vi "AB_Engine_AddExportClassInfo.vi"(8 "ClassInfo":T1[](array[typedef]), 10 "DataTypes":string[](array[string]), 11 "ExportClassInfo":T1[](array[typedef])) -> (3 "ExportClassInfoOut":T1[](array[typedef]))   [LabVIEW 2020]
uses:
  <vilib>/AppBuilder/AB_InteropAssembly_DistVI_Class_Info.ctl
  <vilib>/AppBuilder/IOStatus.ctl
  <vilib>/xml/Close Reference(Node).vi
  <vilib>/xml/NI_XML.lvlib
  <resource>/objmgr/DOMUserDefRef.rc
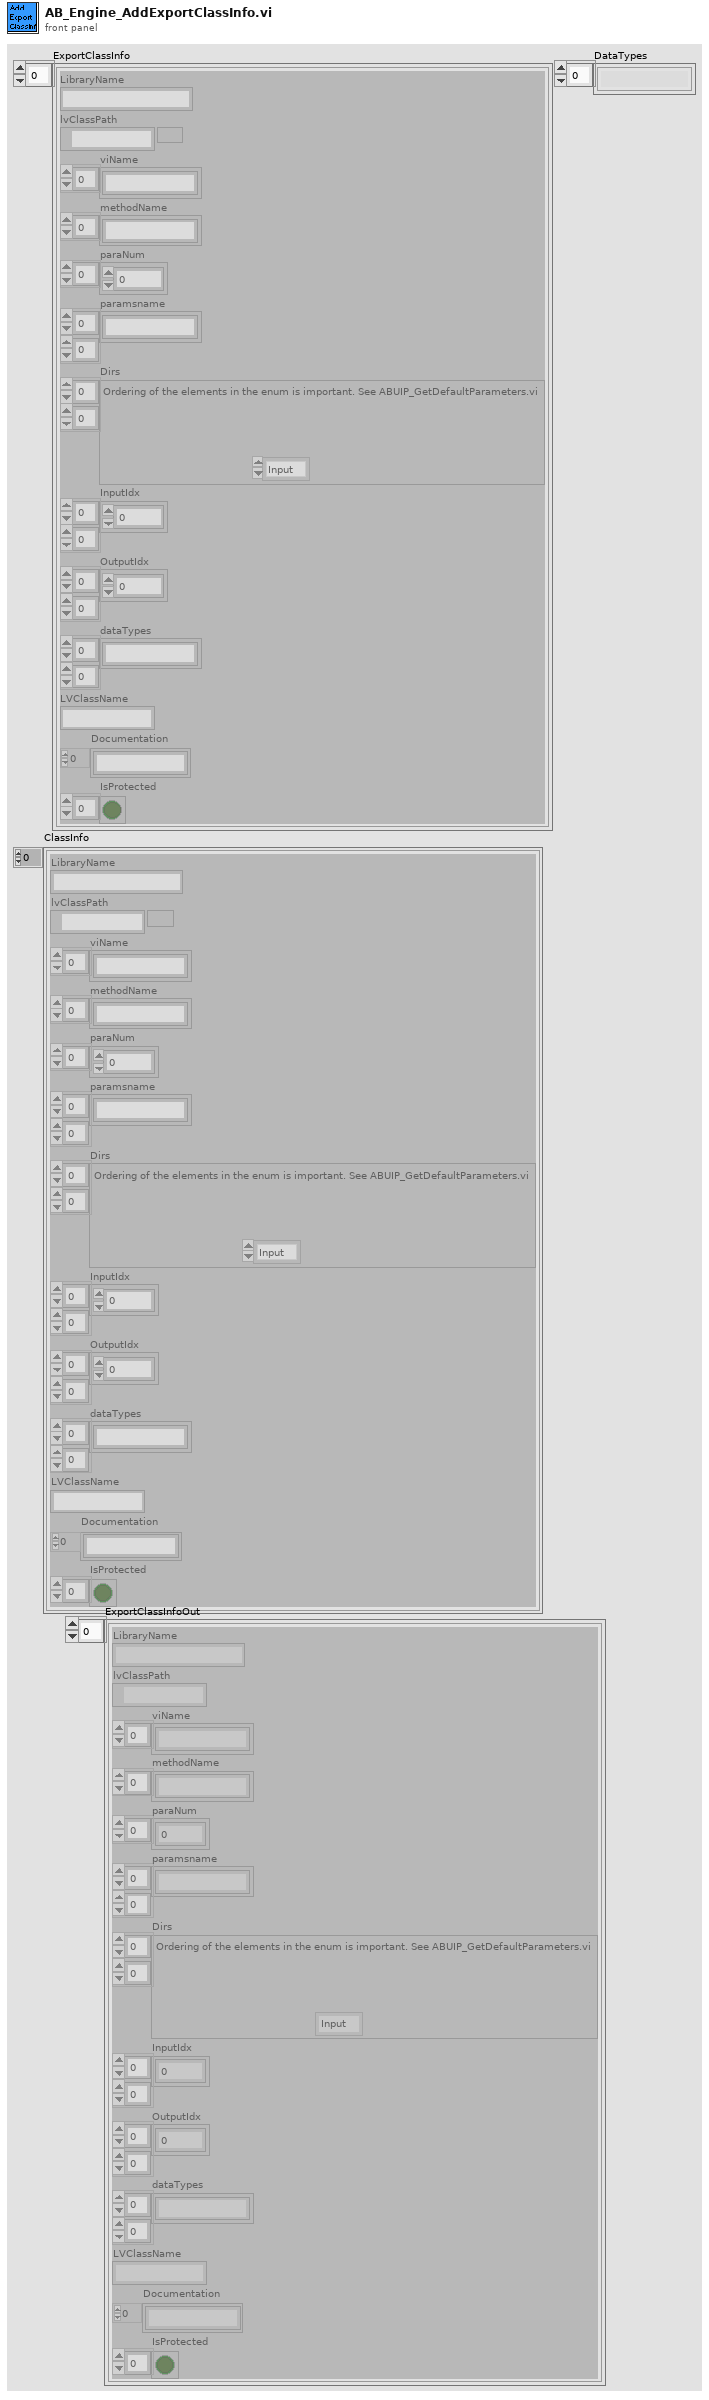
[diagram p1: front panel]
types:
  T1 = typedef "AB_InteropAssembly_DistVI_Class_Info.ctl" = cluster{"LibraryName":string, "lvClassPath":path, "viName":string[], "methodName":string[], "paraNum":i32[], "paramsname":string[][], "Dirs":T2[][], "InputIdx":i32[][], "OutputIdx":i32[][], "dataTypes":string[][], "LVClassName":string, "Documentation":string[], "IsProtected":bool[]}
  T2 = typedef "IOStatus.ctl" = enum16{"Input", "Output", "Input/Output", "InputDeleted", "OutputDeleted", "IODeleted", "ErrorClusterIn", "ErrorClusterOut"}
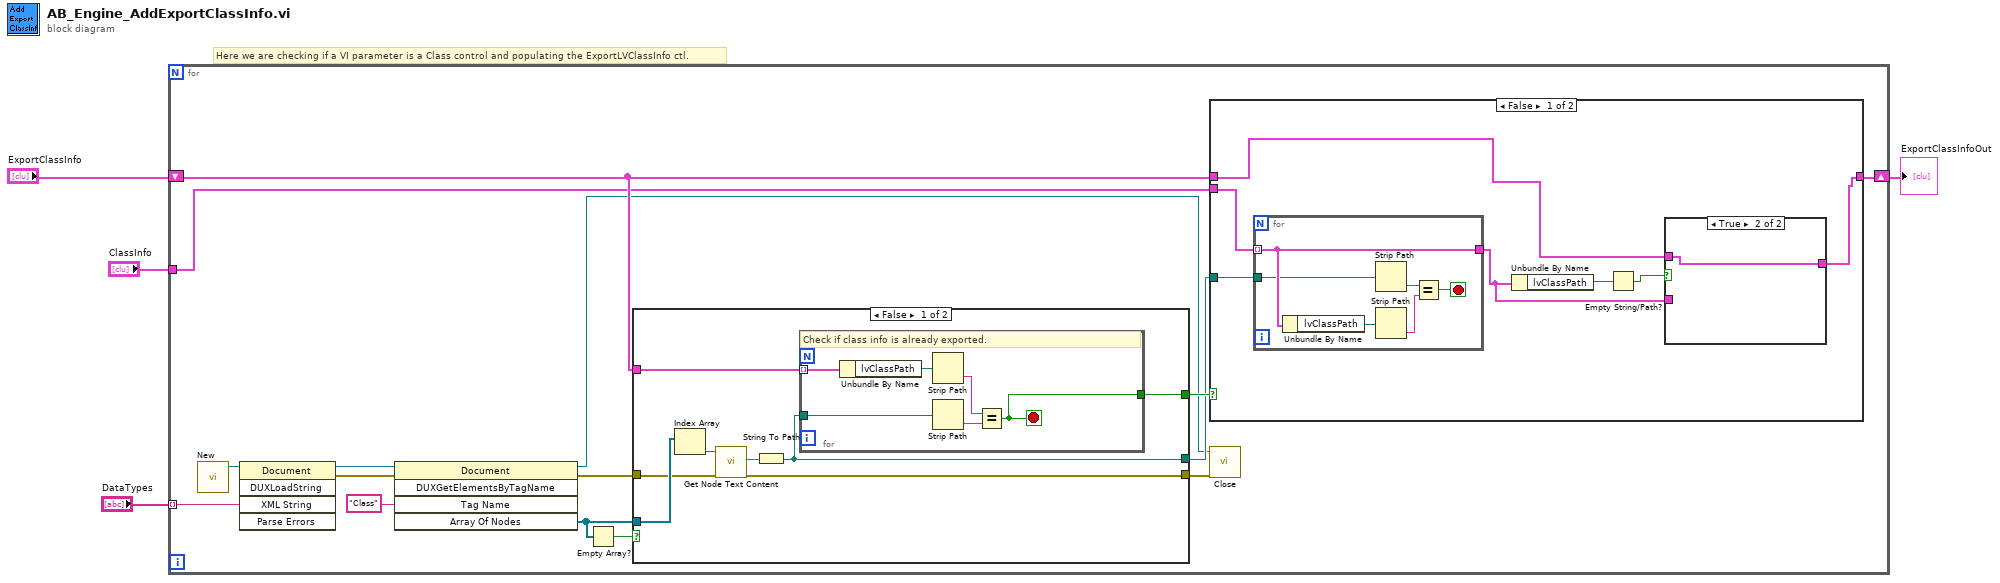
[diagram p0: block diagram]
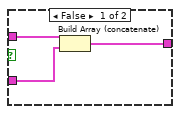
[diagram p2: hidden frame]
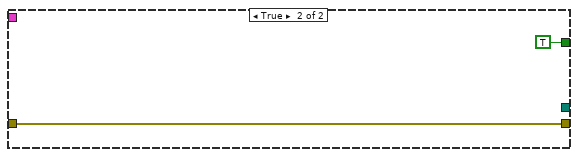
[diagram p4: hidden frame]
diagram:
  # "Here we are checking if a VI parameter is a Class control and populating the ExportLVClassInfo ctl."
  n1 = for {
    tunnel: "DataTypes" -> [w19] mode=indexing
    shift-right: [w10] -> w1
    shift-left: "ExportClassInfo" -> [w12]
    tunnel: "ClassInfo" -> [w5]
    n2 = call <vilib>:"New.vi"() -> ("DOM document out"=w18:refnum<k20>)  [unwired: 1 in, 8 out]
    n3 = invoke class="Document" method="DUXLoadString"(reference=w18, "XML String"=w19) -> (reference out=w17:refnum<k20>, error out=w9:errorcluster)  [unwired: 3 in, 3 out]
    n4 = invoke class="Document" method="DUXGetElementsByTagName"(reference=w17, error in=w9, "Tag Name"="Class") -> (reference out=w6:refnum<k20>, error out=w8:errorcluster, "Array Of Nodes"=w14:refnum<k20>[])  [unwired: 2 in, 2 out]
    n5 = Empty Array?(array=w14) -> (empty?=w15:bool)
    n6 = case shown="False" w15 {
      tunnel: w14 -> [w45 _]
      tunnel: w12 -> [w44 _]
      tunnel: [w43 TRUE] -> w13
      tunnel: [w38 _] -> w11
      tunnel: w8 -> [w40 w53]
      tunnel: [w39 w53] -> w7
      frame False {
        n7 = Index Array(array=w45) -> (element=w42:refnum<k20>)  [unwired: 1 in]
        n8 = call <vilib>:"Get Node Text Content.vi"("error in (no error)"=w40, "node in"=w42) -> ("error out"=w39:errorcluster, "node text"=w41:string)  [unwired: 8 out]
        n9 = String To Path(string=w41) -> (path=w38:path)
        n10 = for {
          tunnel: w44 -> [w51] mode=indexing
          tunnel: w38 -> [w47]
          tunnel: [w50] -> w43
          stop <- w50 stop-if-true
          # "Check if class info is already exported."
          n11 = Unbundle By Name(w51) -> ("lvClassPath"=w49:path)
          n12 = Strip Path(path=w49) -> (name=w48:string)  [unwired: 1 out]
          n13 = Strip Path(path=w47) -> (name=w46:string)  [unwired: 1 out]
          n14 = Equal?(x=w48, y=w46) -> (x = y?=w50:bool)
        }
      }
      frame True {
      }
    }
    n15 = case shown="False" w13 {
      tunnel: w12 -> [w22 w37]
      tunnel: [w20 w37] -> w10
      tunnel: w11 -> [w25 _]
      tunnel: w5 -> [w26 _]
      frame False {
        n16 = for {
          tunnel: w26 -> [w35] mode=indexing
          tunnel: w25 -> [w32]
          tunnel: [w35] -> w21
          stop <- w36 stop-if-true
          n17 = Unbundle By Name(w35) -> ("lvClassPath"=w34:path)
          n18 = Strip Path(path=w32) -> (name=w31:string)  [unwired: 1 out]
          n19 = Strip Path(path=w34) -> (name=w33:string)  [unwired: 1 out]
          n20 = Equal?(x=w31, y=w33) -> (x = y?=w36:bool)
        }
        n21 = Unbundle By Name(w21) -> ("lvClassPath"=w24:path)
        n22 = Empty String/Path?(string/path=w24) -> (empty?=w23:bool)
        n23 = case shown="True" w23 {
          tunnel: w22 -> [w28 w30]
          tunnel: w21 -> [w29 _]
          tunnel: [w27 w30] -> w20
          frame False {
            n24 = Build Array (concatenate)(w28, w29) -> (w27:T1[])
          }
          frame True {
          }
        }
      }
      frame True {
      }
    }
    n25 = call-poly <vilib>:"Close.vi"("error in (no error)"=w7, "node"=w6) -> ()  [unwired: 8 out]
  }
  "ExportClassInfoOut" <- w1
